vi "Splash Screen.vi"() -> ()   [LabVIEW 2021]
uses:
  Launcher/launcher.lvclass
  C:/Program Files (x86)/National Instruments/LabVIEW 2021/user.lib/S2 Labs/Module Framework/Modules/Base/Module.lvclass
  <userlib>/S2 Labs/Module Framework/Modules/Base/Splash Status.ctl
  <userlib>/S2 Labs/Module Framework/Modules/Base/Child Ack.ctl
  <userlib>/S2 Labs/Queued State Machine/QSM.lvclass
  4c048de5-f4c0-4df9-8309-0434289039a5.vi
  1b3ca67f-db92-4dcc-b3f4-64e43358b04d.vi
  05bd3b53-cd47-4e1a-baa1-f3c1d51b1487.vi
  de52d0f8-5d65-4044-95e7-29fc7499fbca.vi
  79034520-c28d-4f0c-9a14-0b8b65e89737.vi
  6387db5e-83c7-4a8a-a2fa-863112d48889.vi
  94f245c5-34b8-4d97-a2ba-0bf8ba9ded74.vi
  <userlib>/S2 Labs/Error Reporting/Transport_WinDebug/Transport_WinDebug.lvclass
  C:/Program Files (x86)/National Instruments/LabVIEW 2021/user.lib/S2 Labs/Error Reporting/Transport Class/Transport.lvclass
  <userlib>/S2 Labs/Error Reporting/ER Global.vi
  <userlib>/S2 Labs/Error Reporting/Error Reporting Class/subVIs/Report Error.vi
  <vilib>/Utility/error.llb/Error Cluster From Error Code.vi
  <vilib>/JDP Science/JSONtext/Variant to JSON Text.vi
  <vilib>/JDP Science/JSONtext/LVClass Serializer/JSONtext LVClass Serializer.lvclass
  <userlib>/S2 Labs/Error Reporting/Error Reporting.lvlib
  <userlib>/S2 Labs/Error Reporting/Transport_System/Transport_System.lvclass
  <userlib>/S2 Labs/Module Framework/Modules/Base/Module.lvclass
panel:
  in  "Shutdown":bool
  out "Status":string
  out "Version":string
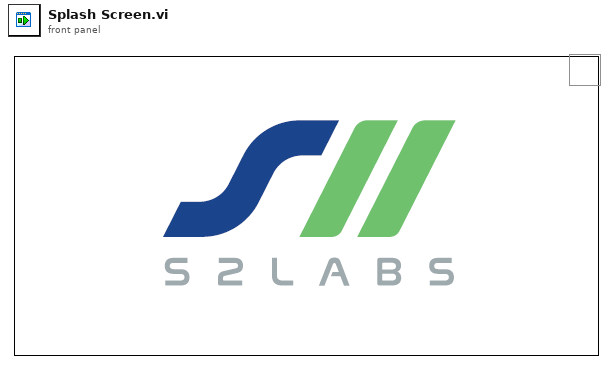
[diagram p1: front panel]
types:
  T1 = typedef "Module.lvclass/Splash Status.ctl" = cluster{"Module Name":string, "Initialized?":bool}
  T2 = enum32{"Invalid", "Standard", "Closed", "Hidden", "Minimized", "Maximized"}
  T3 = typedef "Module.lvclass/Child Ack.ctl" = cluster{"Module Name":string, "Queue":refnum<class "QSM.lvclass">}
  T4 = typedef "QSM.lvclass/Queue Message.ctl" = cluster{"State":T5, "Command":string, "Parameter":variant}
  T5 = typedef "QSM.lvclass/States.ctl" = enum16{"Waiting", "Init", "ExecCMD", "Read Config", "Write Config", "Launch", "Connect", "Recovery", "Clean Up", "Exit"}
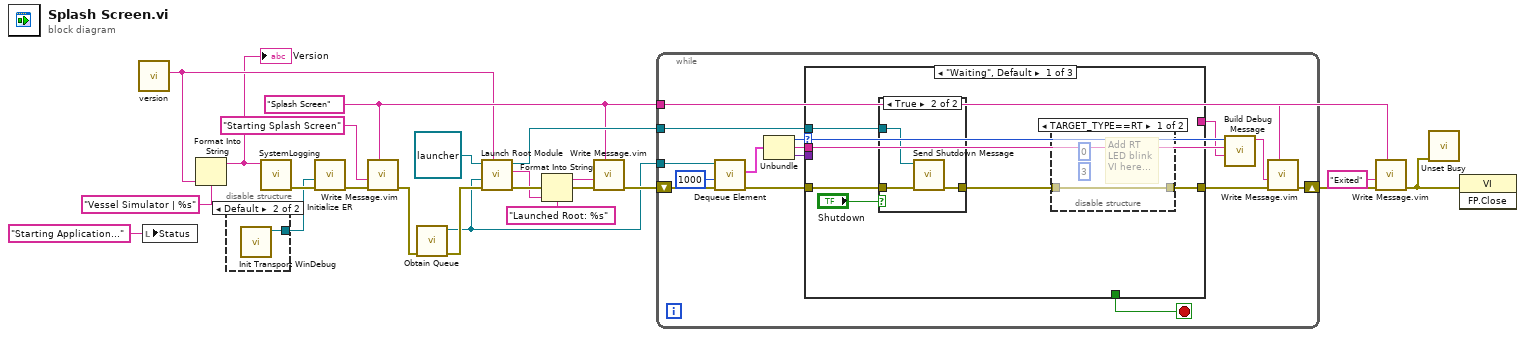
[diagram p0: block diagram]
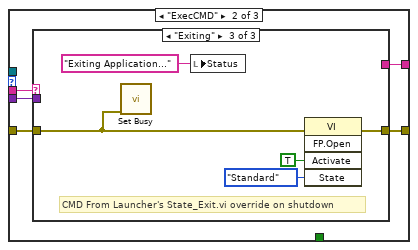
[diagram p4: hidden frame]
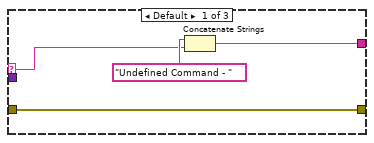
[diagram p5: hidden frame]
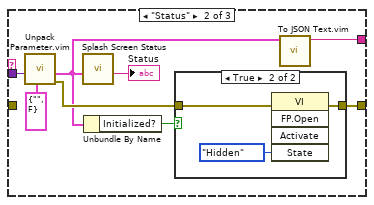
[diagram p6: hidden frame]
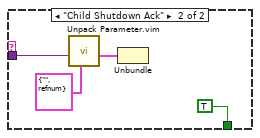
[diagram p9: hidden frame]
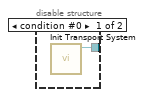
[diagram p10: hidden frame]
diagram:
  w7 = "Splash Screen" ("Message Tag")
  n1 = call "version.vi"() -> ("version"=w4:string)  [unwired: 11 in]
  n2 = local write "Status"("Starting Application..." ("Status")) -> ()
  n3 = Format Into String(format string="Vessel Simulator | %s" ("message"), w4) -> (resulting string=w3:string)  [unwired: 2 in, 1 out]
  "Version" <- w3
  n4 = disable-structure shown="Default" {
    disable-tunnel: [w23 w24] -> w13
    frame condition #0 {
      n5 = call <userlib>:"Init Transport System.vi"() -> ("Transport System"=w23:refnum<class "Transport_System.lvclass">)  [unwired: 11 in]
    }
    frame condition #1 (active) {
      n6 = call <userlib>:"Init Transport WinDebug.vi"() -> ("Transport WinDebug"=w24:refnum<class "Transport_WinDebug.lvclass">)  [unwired: 11 in]
    }
  }
  n7 = call <userlib>:"SystemLogging.vi"("message"=w3) -> ("error out"=w22:errorcluster)  [unwired: 10 in]
  n8 = call <userlib>:"Initialize ER.vi"("error in (no error)"=w22, "Transport Class (UDP)"=w13) -> ("error out"=w21:errorcluster)  [unwired: 9 in]
  n9 = call "Write Message.vim"("Message Tag"=w7, "error in (no error)"=w21, "Message (string)"="Starting Splash Screen") -> ("error out"=w12:errorcluster)  [unwired: 8 in]
  n10 = call <userlib>:"Obtain Queue.vi"("error in (no error)"=w12) -> ("error out"=w11:errorcluster, "QSM"=w9:refnum<class "QSM.lvclass">)  [unwired: 8 in, 1 out]
  n11 = call <userlib>:"Launch Root Module.vi"("App Version"=w4, "error in (no error)"=w11, "Caller Queue"=w9, "Module In"=refnum<class "launcher.lvclass"> refnum ("shell.lvclass")) -> ("error out"=w19:errorcluster, "Name"=w18:string, "Queue Out"=w10:refnum<class "QSM.lvclass">)  [unwired: 5 in]
  n12 = Format Into String(format string="Launched Root: %s", w18) -> (resulting string=w16:string)  [unwired: 2 in, 1 out]
  n13 = call "Write Message.vim"("Message Tag"=w7, "error in (no error)"=w19, "Message (string)"=w16) -> ("error out"=w15:errorcluster)  [unwired: 8 in]
  n14 = while {
    shift-right: [w30] -> w8
    shift-left: w15 -> [w37]
    tunnel: w9 -> [w38]
    tunnel: w10 -> [w34]
    tunnel: w7 -> [w29]
    stop <- w32 stop-if-true
    n15 = call <userlib>:"Dequeue Element.vi"("error in (no error)"=w37, "timeout in ms (-1)"=1000, "QSM in"=w38) -> ("error out"=w36:errorcluster, "Message"=w35:T4)  [unwired: 3 in, 4 out]
    n16 = Unbundle(w35) -> ("State"=w28:T5, "Command"=w27:string, "Parameter"=w33:variant)
    n17 = case shown="\"Waiting\", Default" w28 {
      tunnel: w36 -> [w41 w52 w80]
      tunnel: w34 -> [w43 _ _]
      tunnel: w27 -> [_ w55 w77]
      tunnel: w33 -> [_ w54 w78]
      tunnel: [w44 w53 w80] -> w31
      tunnel: [_ _ w79] -> w32
      tunnel: [_ w51 _] -> w26
      frame "Waiting", Default {
        n18 = case shown="True" "Shutdown" {
          tunnel: w43 -> [_ w48]
          tunnel: w41 -> [w45 w46]
          tunnel: [w45 w47] -> w40
          frame False {
          }
          frame True {
            n19 = call <userlib>:"Send Shutdown Message.vi"("error in (no error)"=w46, "Queue Ref"=w48) -> ("error out"=w47:errorcluster)  [unwired: 9 in]
          }
        }
        n20 = disable-structure shown="TARGET_TYPE==RT" {
          disable-tunnel: w40 -> [w49 w50]
          disable-tunnel: [w49 w50] -> w44
          frame condition #0 {
            (unwired) 3 ("State")
            (unwired) 0 ("LED Num")
            # "Add RT\nLED blink\nVI here..."
          }
          frame condition #1 (active) {
          }
        }
      }
      frame "ExecCMD" {
        n21 = case shown="\"Exiting\"" w55 {
          selector: w55 -> [w56 _ _]
          tunnel: w54 -> [_ w67 _]
          tunnel: [w59 w62 w73] -> w53
          tunnel: w52 -> [w59 _ w72]
          tunnel: [w58 w64 _] -> w51
          frame Default {
            n22 = Concatenate Strings("Undefined Command - ", w56) -> (w58:string)
          }
          frame "Status" {
            n23 = call "Unpack Parameter.vim"("Parameter type (string)"=T1 {"Module Name"="", "Initialized?"=FALSE}, "Parameter Variant"=w67) -> ("error out"=w61:errorcluster, "Parameter"=w60:T1)  [unwired: 8 in]
            n24 = call <userlib>:"Splash Screen Status.vi"("Status Message"=w60) -> ("Status"=→"Status":string)  [unwired: 10 in]
            n25 = Unbundle By Name(w60) -> ("Initialized?"=w63:bool)
            n26 = case shown="True" w63 {
              tunnel: w61 -> [w68 w71]
              tunnel: [w68 w70] -> w62
              frame False {
              }
              frame True {
                n27 = invoke class="VI" method="FP.Open"(error in=w71, "State"=T2."Hidden") -> (error out=w70:errorcluster)  [unwired: 3 in, 4 out]
              }
            }
            n28 = call "To JSON Text.vim"("Anything"=w60) -> ("<JSON>"=w64:string)  [unwired: 9 in, 1 out]
          }
          frame "Exiting" {
            # "CMD From Launcher's State_Exit.vi override on shutdown"
            n29 = call <vilib>:"Set Busy.vi"("error in (no error)"=w72) -> ()  [unwired: 9 in, 2 out]
            n30 = local write "Status"("Exiting Application..." ("Status")) -> ()
            n31 = invoke class="VI" method="FP.Open"(error in=w72, "Activate"=TRUE ("Activate?"), "State"=T2."Standard") -> (error out=w73:errorcluster)  [unwired: 2 in, 4 out]
          }
        }
      }
      frame "Exit" {
        n32 = case shown="Default" w77 {
          tunnel: [_ TRUE] -> w79
          tunnel: w78 -> [_ w83]
          frame Default {
          }
          frame "Child Shutdown Ack" {
            n33 = call "Unpack Parameter.vim"("Parameter type (string)"=T3 {"Module Name"="", "Queue"=refnum} ("Child Ack"), "Parameter Variant"=w83) -> ("Parameter"=w82:T3)  [unwired: 8 in, 1 out]
            n34 = Unbundle(w82) -> ()  [unwired: 2 out]
          }
        }
      }
    }
    n35 = call <userlib>:"Build Debug Message.vi"("Debug Message"=w26, "Command"=w27, "State"=w28) -> ("Built Message"=w25:string)  [unwired: 8 in]
    n36 = call "Write Message.vim"("Message Tag"=w29, "error in (no error)"=w31, "Message (string)"=w25) -> ("error out"=w30:errorcluster)  [unwired: 8 in]
  }
  n37 = call "Write Message.vim"("Message Tag"=w7, "error in (no error)"=w8, "Message (string)"="Exited") -> ("error out"=w1:errorcluster)  [unwired: 8 in]
  n38 = call <vilib>:"Unset Busy.vi"("error in (no error)"=w1) -> ()  [unwired: 10 in, 1 out]
  n39 = invoke class="VI" method="FP.Close"(error in=w1) -> ()  [unwired: 2 in, 3 out]
